vi "Set Setpoint.vi"(10 "setpoint":dbl, 11 "PIDClass.lvclass":refnum<class "PIDClass.lvclass">) -> (3 "PIDClass.lvclass out":refnum<class "PIDClass.lvclass">)   [LabVIEW 2011, in "PIDClass.lvclass"]
uses:
  PIDClass.lvclass
  PIDClass.lvclass/PIDClass.ctl
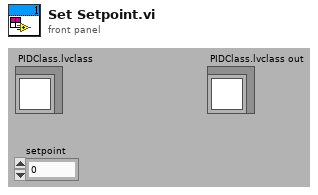
[diagram p1: front panel]
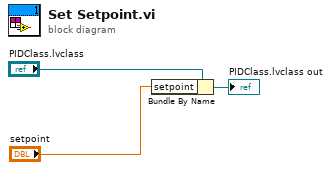
[diagram p0: block diagram]
diagram:
  n1 = Bundle By Name(cluster="PIDClass.lvclass", "setpoint"="setpoint") -> (→"PIDClass.lvclass out":refnum<class "PIDClass.lvclass">)
